vi "Read Full Configuration File.vi"(7 "Config File Path":path) -> (4 "Unique Notifier Names":string[](array[string]), 8 "Device Port/ID/Channel Info":string[][](array[string]), 13 "Configuration Name":string, 15 "Device Engine Paths":path[](array[path]))   [LabVIEW 2020]
panel:
  out "File Lines":string[](array[string])
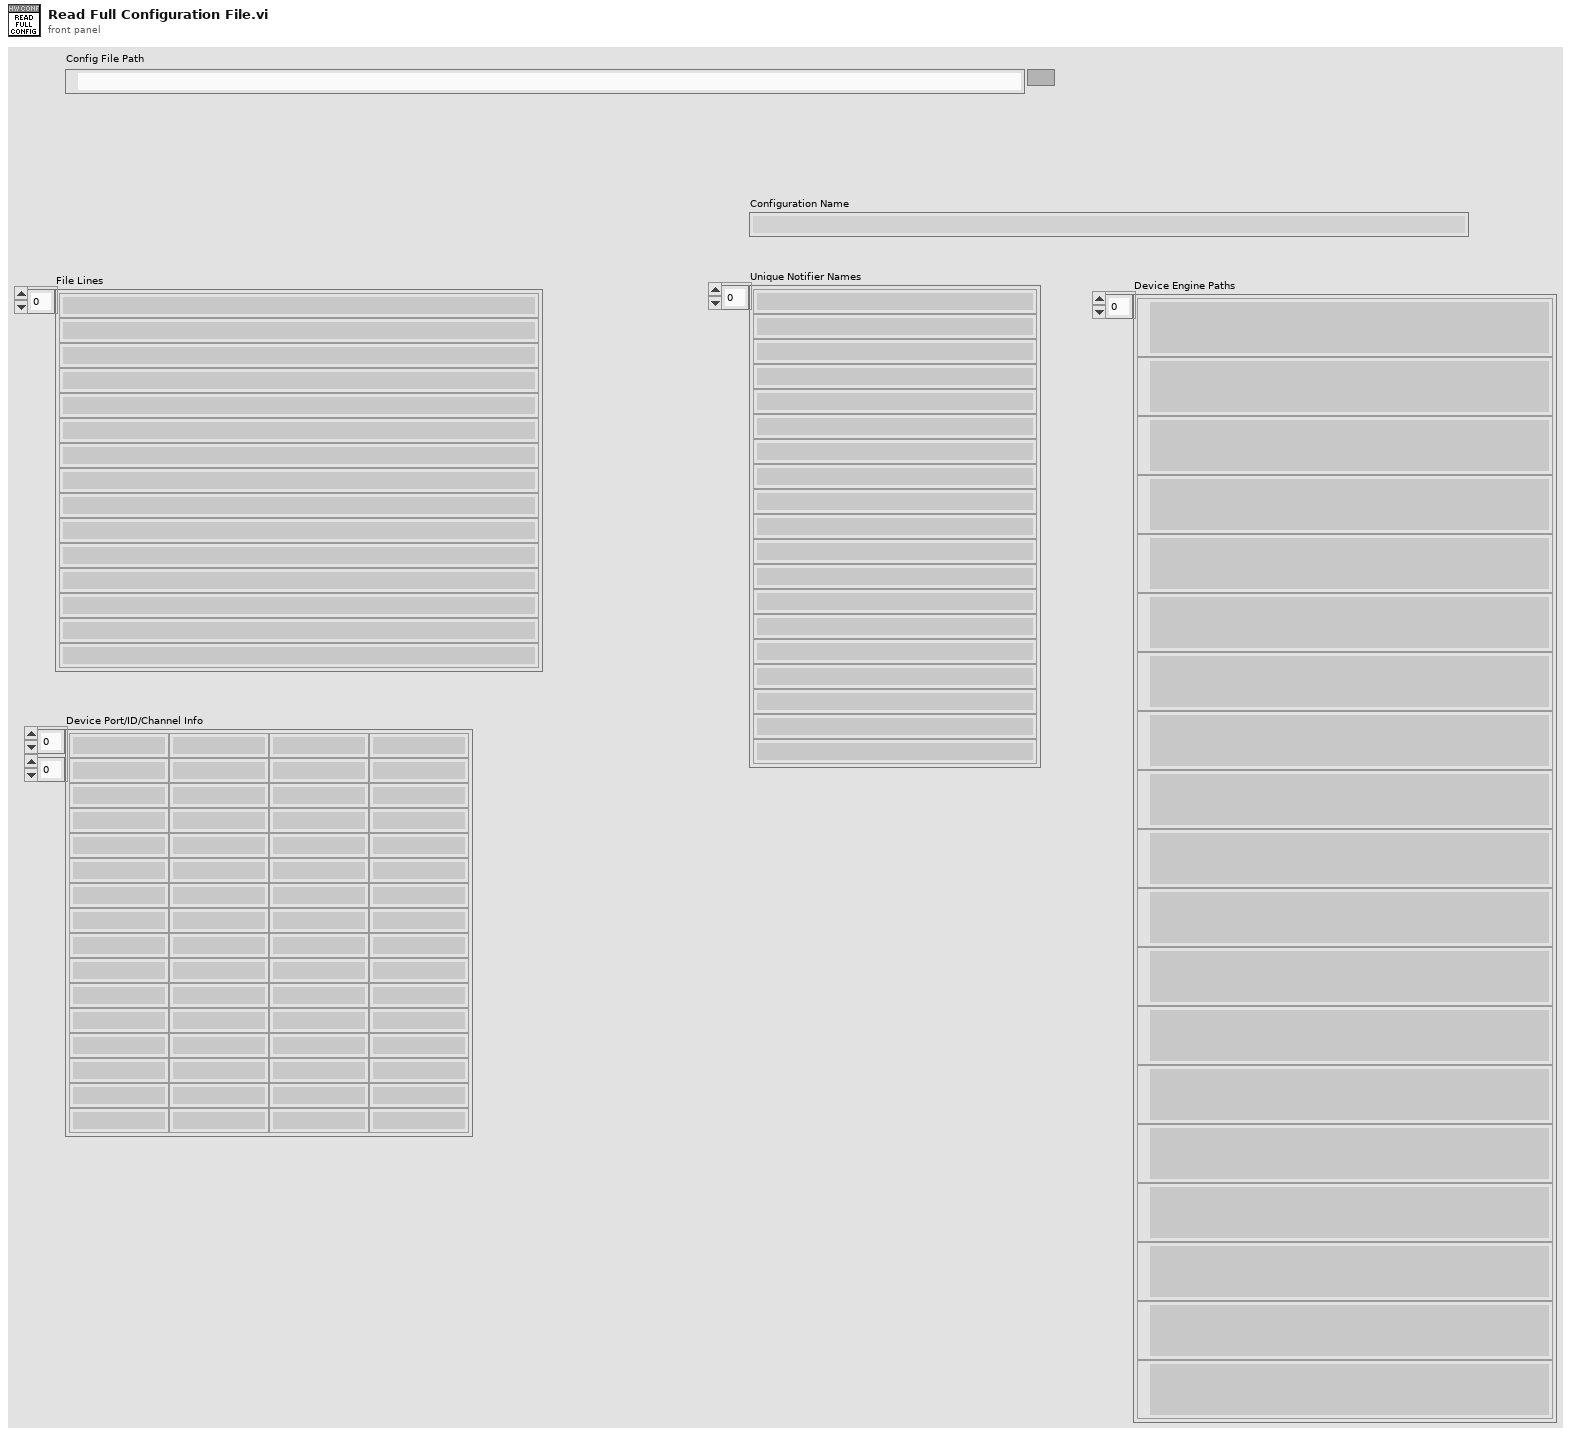
[diagram p1: front panel]
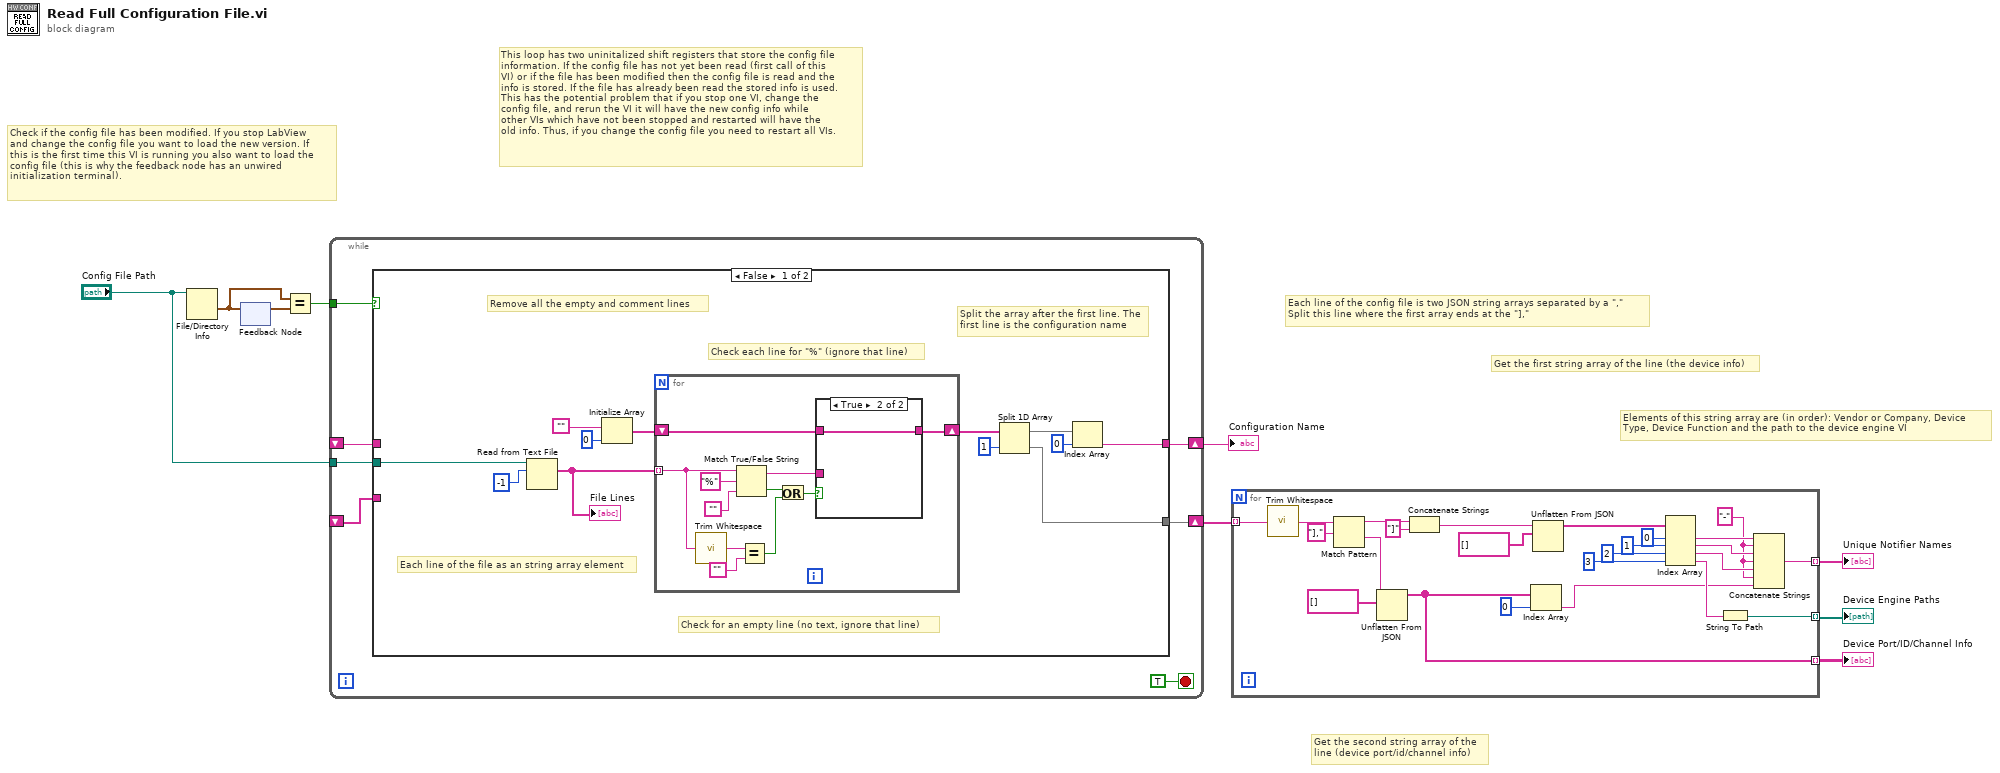
[diagram p0: block diagram]
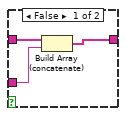
[diagram p2: hidden frame]
diagram:
  # "Get the second string array of the\nline (device port/id/channel info)"
  # "Get the first string array of the line (the device info)"
  # "Each line of the config file is two JSON string arrays separated by a \",\"\nSplit this line where the first array ends at the \"],\""
  # "Elements of this string array are (in order): Vendor or Company, Device\nType, Device Function and the path to the device engine VI"
  # "This loop has two uninitalized shift registers that store the config file\ninformation. If the config file has not yet been read (first call of this\nVI) or if the file has been modified then the config file is read and the\ninfo is stored. If the file has already been read the stored info is used.\nThis has the potential problem that if you stop one VI, change the\nconfig file, and rerun the VI it will have the new config info while\nother VIs which have not been stopped and restarted will have the\nold info. Thus, if you change the config file you need to restart all VIs."
  # "Check if the config file has been modified. If you stop LabView\nand change the config file you want to load the new version. If\nthis is the first time this VI is running you also want to load the\nconfig file (this is why the feedback node has an unwired\ninitialization terminal)."
  n1 = File/Directory Info(path="Config File Path") -> (last mod=w7:timestamp)  [unwired: 1 in, 6 out]
  n2 = feedback-in #1(w7) -> ()
  n3 = feedback #1() -> (w8:timestamp)  [unwired: 1 in]
  n4 = Equal?(x=w7, y=w8) -> (x = y?=w6:bool)
  n5 = while {
    shift-right: [w15] -> w4
    shift-left: _ -> [w12]
    shift-right: [w16] -> w9
    shift-left: _ -> [w13]
    tunnel: w6 -> [w11]
    tunnel: "Config File Path" -> [w10]
    stop <- TRUE stop-if-true
    n6 = case shown="False" w11 {
      tunnel: [w19 w45] -> w16
      tunnel: [w18 w44] -> w15
      tunnel: w13 -> [_ w45]
      tunnel: w12 -> [_ w44]
      tunnel: w10 -> [w17 _]
      frame False {
        # "Split the array after the first line. The\nfirst line is the configuration name"
        # "Remove all the empty and comment lines"
        # "Each line of the file as an string array element"
        # "Check for an empty line (no text, ignore that line)"
        # "Check each line for \"%\" (ignore that line)"
        n7 = Read from Text File(file (use dialog)=w17, count=-1) -> (text=w27:string[])  [unwired: 2 in, 3 out]
        "File Lines" <- w27
        n8 = Initialize Array("", 0 ("dimension size")) -> (w24:string[])
        n9 = for {
          tunnel: w27 -> [w34] mode=indexing
          shift-right: [w36] -> w23
          shift-left: w24 -> [w37]
          n10 = call <vilib>:"Trim Whitespace.vi"("string"=w34) -> ("trimmed string"=w33:string)  [unwired: 1 in]
          n11 = Match True/False String(2:"", 3:"%" ("true string"), 4:w34) -> (0:w31:bool, 1:w38:string)
          n12 = Equal?(x=w33, y="") -> (x = y?=w30:bool)
          n13 = Or(x=w31, y=w30) -> (x .or. y?=w29:bool)
          n14 = case shown="True" w29 {
            tunnel: w38 -> [w40 _]
            tunnel: w37 -> [w42 w43]
            tunnel: [w41 w43] -> w36
            frame False {
              n15 = Build Array (concatenate)(w42, w40) -> (w41:string[])
            }
            frame True {
            }
          }
        }
        n16 = Split 1D Array(array=w23, index=1) -> (first subarray=w21:string[], second subarray=w18:string[])
        n17 = Index Array(array=w21, index=0) -> (element=w19:string)
      }
      frame True {
      }
    }
  }
  "Configuration Name" <- w9
  n18 = for {
    tunnel: w4 -> [w51] mode=indexing
    tunnel: [w50] -> w3 mode=indexing
    tunnel: [w49] -> w2 mode=indexing
    tunnel: [w46] -> w1 mode=indexing
    w52 = "-"
    n19 = call <vilib>:"Trim Whitespace.vi"("string"=w51) -> ("trimmed string"=w68:string)  [unwired: 1 in]
    n20 = Match Pattern(string=w68, regular expression="],") -> (before substring=w67:string, after substring=w64:string)  [unwired: 1 in, 2 out]
    n21 = Unflatten From JSON(JSON string=w64, type and defaults=string[] []) -> (value=w46:string[])  [unwired: 5 in, 1 out]
    n22 = Concatenate Strings(w67, "]" ("string")) -> (w65:string)
    n23 = Index Array(array=w46, index=0) -> (element=w48:string)
    n24 = Unflatten From JSON(JSON string=w65, type and defaults=string[] []) -> (value=w61:string[])  [unwired: 5 in, 1 out]
    n25 = Index Array(array=w61, index #1=0 ("index"), index #2=1 ("index"), index #3=2 ("index"), index #4=3 ("index")) -> (element #1=w55:string, element #2=w54:string, element #3=w53:string, element #4=w56:string)
    n26 = String To Path(string=w56) -> (path=w49:path)
    n27 = Concatenate Strings(w55, w52, w54, w52, w53, w52, w48) -> (w50:string)
  }
  "Unique Notifier Names" <- w3
  "Device Engine Paths" <- w2
  "Device Port/ID/Channel Info" <- w1
